vi "test TCX read (installed 71).vi"() -> ()   [LabVIEW 2011] (continued)
ackpoint><Time>2008-03-03T23:06:16Z</Time><Position><LatitudeDegrees>35.865661</LatitudeDegrees><LongitudeDegrees>-78.879918</LongitudeDegrees></Position><AltitudeMeters>73.678</AltitudeMeters><DistanceMeters>11620.606</DistanceMeters><Cadence>66</Cadence><Extensions><TPX xmlns=\"http://www.garmin.com/xmlschemas/ActivityExtension/v2\"><Watts>364</Watts></TPX></Extensions></Trackpoint><Trackpoint><Time>2008-03-03T23:06:17Z</Time><Position><LatitudeDegrees>35.865731</LatitudeDegrees><LongitudeDegrees>-78.879935</LongitudeDegrees></Position><AltitudeMeters>73.678</AltitudeMeters><DistanceMeters>11628.598</DistanceMeters><Cadence>65</Cadence><Extensions><TPX xmlns=\"http://www.garmin.com/xmlschemas/ActivityExtension/v2\"><Watts>362</Watts></TPX></Extensions></Trackpoint><Trackpoint><Time>2008-03-03T23:06:18Z</Time><Position><LatitudeDegrees>35.865801</LatitudeDegrees><LongitudeDegrees>-78.879955</LongitudeDegrees></Position><AltitudeMeters>73.678</AltitudeMeters><DistanceMeters>11636.497</DistanceMeters><Cadence>65</Cadence><Extensions><TPX xmlns=\"http://www.garmin.com/xmlschemas/ActivityExtension/v2\"><Watts>356</Watts></TPX></Extensions></Trackpoint><Trackpoint><Time>2008-03-03T23:06:19Z</Time><Position><LatitudeDegrees>35.865870</LatitudeDegrees><LongitudeDegrees>-78.879979</LongitudeDegrees></Position><AltitudeMeters>74.159</AltitudeMeters><DistanceMeters>11644.413</DistanceMeters><Cadence>65</Cadence><Extensions><TPX xmlns=\"http://www.garmin.com/xmlschemas/ActivityExtension/v2\"><Watts>355</Watts></TPX></Extensions></Trackpoint><Trackpoint><Time>2008-03-03T23:06:20Z</Time><Position><LatitudeDegrees>35.865936</LatitudeDegrees><LongitudeDegrees>-78.880009</LongitudeDegrees></Position><AltitudeMeters>74.640</AltitudeMeters><DistanceMeters>11652.265</DistanceMeters><Cadence>64</Cadence><Extensions><TPX xmlns=\"http://www.garmin.com/xmlschemas/ActivityExtension/v2\"><Watts>312</Watts></TPX></Extensions></Trackpoint><Trackpoint><Time>2008-03-03T23:06:21Z</Time><Position><LatitudeDegrees>35.866001</LatitudeDegrees><LongitudeDegrees>-78.880044</LongitudeDegrees></Position><AltitudeMeters>74.640</AltitudeMeters><DistanceMeters>11660.149</DistanceMeters><Cadence>64</Cadence><Extensions><TPX xmlns=\"http://www.garmin.com/xmlschemas/ActivityExtension/v2\"><Watts>275</Watts></TPX></Extensions></Trackpoint><Trackpoint><Time>2008-03-03T23:06:22Z</Time><Position><LatitudeDegrees>35.866066</LatitudeDegrees><LongitudeDegrees>-78.880082</LongitudeDegrees></Position><AltitudeMeters>74.640</AltitudeMeters><DistanceMeters>11668.127</DistanceMeters><Cadence>64</Cadence><Extensions><TPX xmlns=\"http://www.garmin.com/xmlschemas/ActivityExtension/v2\"><Watts>233</Watts></TPX></Extensions></Trackpoint><Trackpoint><Time>2008-03-03T23:06:23Z</Time><Position><LatitudeDegrees>35.866131</LatitudeDegrees><LongitudeDegrees>-78.880120</LongitudeDegrees></Position><AltitudeMeters>74.640</AltitudeMeters><DistanceMeters>11676.109</DistanceMeters><Cadence>65</Cadence><Extensions><TPX xmlns=\"http://www.garmin.com/xmlschemas/ActivityExtension/v2\"><Watts>109</Watts></TPX></Extensions></Trackpoint><Trackpoint><Time>2008-03-03T23:06:24Z</Time><Position><LatitudeDegrees>35.866196</LatitudeDegrees><LongitudeDegrees>-78.880160</LongitudeDegrees></Position><AltitudeMeters>74.640</AltitudeMeters><DistanceMeters>11684.144</DistanceMeters><Cadence>66</Cadence><Extensions><TPX xmlns=\"http://www.garmin.com/xmlschemas/ActivityExtension/v2\"><Watts>66</Watts></TPX></Extensions></Trackpoint><Trackpoint><Time>2008-03-03T23:06:25Z</Time><Position><LatitudeDegrees>35.866260</LatitudeDegrees><LongitudeDegrees>-78.880202</LongitudeDegrees></Position><AltitudeMeters>74.640</AltitudeMeters><DistanceMeters>11692.274</DistanceMeters><Cadence>66</Cadence><Extensions><TPX xmlns=\"http://www.garmin.com/xmlschemas/ActivityExtension/v2\"><Watts>59</Watts></TPX></Extensions></Trackpoint><Trackpoint><Time>2008-03-03T23:06:26Z</Time><Position><LatitudeDegrees>35.866323</LatitudeDegrees><LongitudeDegrees>-78.880250</LongitudeDegrees></Position><AltitudeMeters>74.640</AltitudeMeters><DistanceMeters>11700.427</DistanceMeters><Cadence>66</Cadence><Extensions><TPX xmlns=\"http://www.garmin.com/xmlschemas/ActivityExtension/v2\"><Watts>59</Watts></TPX></Extensions></Trackpoint><Trackpoint><Time>2008-03-03T23:06:27Z</Time><Position><LatitudeDegrees>35.866380</LatitudeDegrees><LongitudeDegrees>-78.880308</LongitudeDegrees></Position><AltitudeMeters>74.640</AltitudeMeters><DistanceMeters>11708.690</DistanceMeters><Cadence>68</Cadence><Extensions><TPX xmlns=\"http://www.garmin.com/xmlschemas/ActivityExtension/v2\"><Watts>59</Watts></TPX></Extensions></Trackpoint><Trackpoint><Time>2008-03-03T23:06:28Z</Time><Position><LatitudeDegrees>35.866422</LatitudeDegrees><LongitudeDegrees>-78.880383</LongitudeDegrees></Position><AltitudeMeters>74.640</AltitudeMeters><DistanceMeters>11716.855</DistanceMeters><Cadence>71</Cadence><Extensions><TPX xmlns=\"http://www.garmin.com/xmlschemas/ActivityExtension/v2\"><Watts>97</Watts></TPX></Extensions></Trackpoint><Trackpoint><Time>2008-03-03T23:06:29Z</Time><Position><LatitudeDegrees>35.866438</LatitudeDegrees><LongitudeDegrees>-78.880474</LongitudeDegrees></Position><AltitudeMeters>75.120</AltitudeMeters><DistanceMeters>11725.147</DistanceMeters><Cadence>71</Cadence><Extensions><TPX xmlns=\"http://www.garmin.com/xmlschemas/ActivityExtension/v2\"><Watts>97</Watts></TPX></Extensions></Trackpoint><Trackpoint><Time>2008-03-03T23:06:30Z</Time><Position><LatitudeDegrees>35.866425</LatitudeDegrees><LongitudeDegrees>-78.880568</LongitudeDegrees></Position><AltitudeMeters>74.640</AltitudeMeters><DistanceMeters>11733.718</DistanceMeters><Cadence>71</Cadence><Extensions><TPX xmlns=\"http://www.garmin.com/xmlschemas/ActivityExtension/v2\"><Watts>199</Watts></TPX></Extensions></Trackpoint><Trackpoint><Time>2008-03-03T23:06:31Z</Time><Position><LatitudeDegrees>35.866393</LatitudeDegrees><LongitudeDegrees>-78.880658</LongitudeDegrees></Position><AltitudeMeters>74.640</AltitudeMeters><DistanceMeters>11742.621</DistanceMeters><Cadence>71</Cadence><Extensions><TPX xmlns=\"http://www.garmin.com/xmlschemas/ActivityExtension/v2\"><Watts>199</Watts></TPX></Extensions></Trackpoint><Trackpoint><Time>2008-03-03T23:06:32Z</Time><Position><LatitudeDegrees>35.866355</LatitudeDegrees><LongitudeDegrees>-78.880747</LongitudeDegrees></Position><AltitudeMeters>75.120</AltitudeMeters><DistanceMeters>11751.724</DistanceMeters><Cadence>73</Cadence><Extensions><TPX xmlns=\"http://www.garmin.com/xmlschemas/ActivityExtension/v2\"><Watts>228</Watts></TPX></Extensions></Trackpoint><Trackpoint><Time>2008-03-03T23:06:33Z</Time><Position><LatitudeDegrees>35.866317</LatitudeDegrees><LongitudeDegrees>-78.880838</LongitudeDegrees></Position><AltitudeMeters>75.120</AltitudeMeters><DistanceMeters>11760.945</DistanceMeters><Cadence>75</Cadence><Extensions><TPX xmlns=\"http://www.garmin.com/xmlschemas/ActivityExtension/v2\"><Watts>280</Watts></TPX></Extensions></Trackpoint><Trackpoint><Time>2008-03-03T23:06:34Z</Time><Position><LatitudeDegrees>35.866279</LatitudeDegrees><LongitudeDegrees>-78.880931</LongitudeDegrees></Position><AltitudeMeters>75.120</AltitudeMeters><DistanceMeters>11770.377</DistanceMeters><Cadence>76</Cadence><Extensions><TPX xmlns=\"http://www.garmin.com/xmlschemas/ActivityExtension/v2\"><Watts>320</Watts></TPX></Extensions></Trackpoint><Trackpoint><Time>2008-03-03T23:06:35Z</Time><Position><LatitudeDegrees>35.866240</LatitudeDegrees><LongitudeDegrees>-78.881024</LongitudeDegrees></Position><AltitudeMeters>75.120</AltitudeMeters><DistanceMeters>11779.813</DistanceMeters><Cadence>76</Cadence><Extensions><TPX xmlns=\"http://www.garmin.com/xmlschemas/ActivityExtension/v2\"><Watts>272</Watts></TPX></Extensions></Trackpoint><Trackpoint><Time>2008-03-03T23:06:36Z</Time><Position><LatitudeDegrees>35.866200</LatitudeDegrees><LongitudeDegrees>-78.881116</LongitudeDegrees></Position><AltitudeMeters>75.120</AltitudeMeters><DistanceMeters>11789.220</DistanceMeters><Cadence>76</Cadence><Extensions><TPX xmlns=\"http://www.garmin.com/xmlschemas/ActivityExtension/v2\"><Watts>270</Watts></TPX></Extensions></Trackpoint><Trackpoint><Time>2008-03-03T23:06:37Z</Time><Position><LatitudeDegrees>35.866164</LatitudeDegrees><LongitudeDegrees>-78.881205</LongitudeDegrees></Position><AltitudeMeters>75.120</AltitudeMeters><DistanceMeters>11798.199</DistanceMeters><Cadence>75</Cadence><Extensions><TPX xmlns=\"http://www.garmin.com/xmlschemas/ActivityExtension/v2\"><Watts>204</Watts></TPX></Extensions></Trackpoint><Trackpoint><Time>2008-03-03T23:06:38Z</Time><Position><LatitudeDegrees>35.866129</LatitudeDegrees><LongitudeDegrees>-78.881295</LongitudeDegrees></Position><AltitudeMeters>75.601</AltitudeMeters><DistanceMeters>11807.172</DistanceMeters><Cadence>73</Cadence><Extensions><TPX xmlns=\"http://www.garmin.com/xmlschemas/ActivityExtension/v2\"><Watts>205</Watts></TPX></Extensions></Trackpoint><Trackpoint><Time>2008-03-03T23:06:39Z</Time><Position><LatitudeDegrees>35.866092</LatitudeDegrees><LongitudeDegrees>-78.881383</LongitudeDegrees></Position><AltitudeMeters>75.601</AltitudeMeters><DistanceMeters>11816.092</DistanceMeters><Cadence>71</Cadence><Extensions><TPX xmlns=\"http://www.garmin.com/xmlschemas/ActivityExtension/v2\"><Watts>231</Watts></TPX></Extensions></Trackpoint><Trackpoint><Time>2008-03-03T23:06:40Z</Time><Position><LatitudeDegrees>35.866055</LatitudeDegrees><LongitudeDegrees>-78.881469</LongitudeDegrees></Position><AltitudeMeters>75.120</AltitudeMeters><DistanceMeters>11824.877</DistanceMeters><Cadence>70</Cadence><Extensions><TPX xmlns=\"http://www.garmin.com/xmlschemas/ActivityExtension/v2\"><Watts>239</Watts></TPX></Extensions></Trackpoint><Trackpoint><Time>2008-03-03T23:06:41Z</Time><Position><LatitudeDegrees>35.866018</LatitudeDegrees><LongitudeDegrees>-78.881553</LongitudeDegrees></Position><AltitudeMeters>75.601</AltitudeMeters><DistanceMeters>11833.483</DistanceMeters><Cadence>70</Cadence><Extensions><TPX xmlns=\"http://www.garmin.com/xmlschemas/ActivityExtension/v2\"><Watts>241</Watts></TPX></Extensions></Trackpoint><Trackpoint><Time>2008-03-03T23:06:42Z</Time><Position><LatitudeDegrees>35.865982</LatitudeDegrees><LongitudeDegrees>-78.881636</LongitudeDegrees></Position><AltitudeMeters>75.601</AltitudeMeters><DistanceMeters>11842.034</DistanceMeters><Cadence>69</Cadence><Extensions><TPX xmlns=\"http://www.garmin.com/xmlschemas/ActivityExtension/v2\"><Watts>250</Watts></TPX></Extensions></Trackpoint><Trackpoint><Time>2008-03-03T23:06:43Z</Time><Position><LatitudeDegrees>35.865947</LatitudeDegrees><LongitudeDegrees>-78.881719</LongitudeDegrees></Position><AltitudeMeters>76.081</AltitudeMeters><DistanceMeters>11850.508</DistanceMeters><Cadence>68</Cadence><Extensions><TPX xmlns=\"http://www.garmin.com/xmlschemas/ActivityExtension/v2\"><Watts>251</Watts></TPX></Extensions></Trackpoint><Trackpoint><Time>2008-03-03T23:06:44Z</Time><Position><LatitudeDegrees>35.865912</LatitudeDegrees><LongitudeDegrees>-78.881803</LongitudeDegrees></Position><AltitudeMeters>76.081</AltitudeMeters><DistanceMeters>11858.958</DistanceMeters><Cadence>68</Cadence><Extensions><TPX xmlns=\"http://www.garmin.com/xmlschemas/ActivityExtension/v2\"><Watts>243</Watts></TPX></Extensions></Trackpoint><Trackpoint><Time>2008-03-03T23:06:45Z</Time><Position><LatitudeDegrees>35.865877</LatitudeDegrees><LongitudeDegrees>-78.881885</LongitudeDegrees></Position><AltitudeMeters>76.081</AltitudeMeters><DistanceMeters>11867.346</DistanceMeters><Cadence>68</Cadence><Extensions><TPX xmlns=\"http://www.garmin.com/xmlschemas/ActivityExtension/v2\"><Watts>240</Watts></TPX></Extensions></Trackpoint><Trackpoint><Time>2008-03-03T23:06:46Z</Time><Position><LatitudeDegrees>35.865843</LatitudeDegrees><LongitudeDegrees>-78.881968</LongitudeDegrees></Position><AltitudeMeters>76.562</AltitudeMeters><DistanceMeters>11875.714</DistanceMeters><Cadence>67</Cadence><Extensions><TPX xmlns=\"http://www.garmin.com/xmlschemas/ActivityExtension/v2\"><Watts>234</Watts></TPX></Extensions></Trackpoint><Trackpoint><Time>2008-03-03T23:06:47Z</Time><Position><LatitudeDegrees>35.865810</LatitudeDegrees><LongitudeDegrees>-78.882051</LongitudeDegrees></Position><AltitudeMeters>76.562</AltitudeMeters><DistanceMeters>11884.056</DistanceMeters><Cadence>68</Cadence><Extensions><TPX xmlns=\"http://www.garmin.com/xmlschemas/ActivityExtension/v2\"><Watts>202</Watts></TPX></Extensions></Trackpoint><Trackpoint><Time>2008-03-03T23:06:48Z</Time><Position><LatitudeDegrees>35.865777</LatitudeDegrees><LongitudeDegrees>-78.882134</LongitudeDegrees></Position><AltitudeMeters>76.562</AltitudeMeters><DistanceMeters>11892.388</DistanceMeters><Cadence>68</Cadence><Extensions><TPX xmlns=\"http://www.garmin.com/xmlschemas/ActivityExtension/v2\"><Watts>201</Watts></TPX></Extensions></Trackpoint><Trackpoint><Time>2008-03-03T23:06:49Z</Time><Position><LatitudeDegrees>35.865744</LatitudeDegrees><LongitudeDegrees>-78.882217</LongitudeDegrees></Position><AltitudeMeters>77.043</AltitudeMeters><DistanceMeters>11900.713</DistanceMeters><Cadence>67</Cadence><Extensions><TPX xmlns=\"http://www.garmin.com/xmlschemas/ActivityExtension/v2\"><Watts>182</Watts></TPX></Extensions></Trackpoint><Trackpoint><Time>2008-03-03T23:06:50Z</Time><Position><LatitudeDegrees>35.865711</LatitudeDegrees><LongitudeDegrees>-78.882300</LongitudeDegrees></Position><AltitudeMeters>76.081</AltitudeMeters><DistanceMeters>11909.103</DistanceMeters><Cadence>68</Cadence><Extensions><TPX xmlns=\"http://www.garmin.com/xmlschemas/ActivityExtension/v2\"><Watts>153</Watts></TPX></Extensions></Trackpoint><Trackpoint><Time>2008-03-03T23:06:51Z</Time><Position><LatitudeDegrees>35.865679</LatitudeDegrees><LongitudeDegrees>-78.882385</LongitudeDegrees></Position><AltitudeMeters>77.043</AltitudeMeters><DistanceMeters>11917.494</DistanceMeters><Cadence>68</Cadence><Extensions><TPX xmlns=\"http://www.garmin.com/xmlschemas/ActivityExtension/v2\"><Watts>134</Watts></TPX></Extensions></Trackpoint><Trackpoint><Time>2008-03-03T23:06:52Z</Time><Position><LatitudeDegrees>35.865650</LatitudeDegrees><LongitudeDegrees>-78.882471</LongitudeDegrees></Position><AltitudeMeters>77.043</AltitudeMeters><DistanceMeters>11925.970</DistanceMeters><Cadence>69</Cadence><Extensions><TPX xmlns=\"http://www.garmin.com/xmlschemas/ActivityExtension/v2\"><Watts>120</Watts></TPX></Extensions></Trackpoint><Trackpoint><Time>2008-03-03T23:06:53Z</Time><Position><LatitudeDegrees>35.865621</LatitudeDegrees><LongitudeDegrees>-78.882559</LongitudeDegrees></Position><AltitudeMeters>76.562</AltitudeMeters><DistanceMeters>11934.501</DistanceMeters><Cadence>70</Cadence><Extensions><TPX xmlns=\"http://www.garmin.com/xmlschemas/ActivityExtension/v2\"><Watts>109</Watts></TPX></Extensions></Trackpoint><Trackpoint><Time>2008-03-03T23:06:54Z</Time><Position><LatitudeDegrees>35.865594</LatitudeDegrees><LongitudeDegrees>-78.882648</LongitudeDegrees></Position><AltitudeMeters>76.081</AltitudeMeters><DistanceMeters>11943.104</DistanceMeters><Cadence>70</Cadence><Extensions><TPX xmlns=\"http://www.garmin.com/xmlschemas/ActivityExtension/v2\"><Watts>103</Watts></TPX></Extensions></Trackpoint><Trackpoint><Time>2008-03-03T23:06:55Z</Time><Position><LatitudeDegrees>35.865566</LatitudeDegrees><LongitudeDegrees>-78.882738</LongitudeDegrees></Position><AltitudeMeters>76.081</AltitudeMeters><DistanceMeters>11951.811</DistanceMeters><Cadence>71</Cadence><Extensions><TPX xmlns=\"http://www.garmin.com/xmlschemas/ActivityExtension/v2\"><Watts>105</Watts></TPX></Extensions></Trackpoint><Trackpoint><Time>2008-03-03T23:06:56Z</Time><Position><LatitudeDegrees>35.865540</LatitudeDegrees><LongitudeDegrees>-78.882830</LongitudeDegrees></Position><AltitudeMeters>76.562</AltitudeMeters><DistanceMeters>11960.656</DistanceMeters><Cadence>71</Cadence><Extensions><TPX xmlns=\"http://www.garmin.com/xmlschemas/ActivityExtension/v2\"><Watts>104</Watts></TPX></Extensions></Trackpoint><Trackpoint><Time>2008-03-03T23:06:57Z</Time><Position><LatitudeDegrees>35.865514</LatitudeDegrees><LongitudeDegrees>-78.882923</LongitudeDegrees></Position><AltitudeMeters>76.081</AltitudeMeters><DistanceMeters>11969.581</DistanceMeters><Cadence>72</Cadence><Extensions><TPX xmlns=\"http://www.garmin.com/xmlschemas/ActivityExtension/v2\"><Watts>93</Watts></TPX></Extensions></Trackpoint><Trackpoint><Time>2008-03-03T23:06:58Z</Time><Position><LatitudeDegrees>35.865489</LatitudeDegrees><LongitudeDegrees>-78.883018</LongitudeDegrees></Position><AltitudeMeters>76.081</AltitudeMeters><DistanceMeters>11978.509</DistanceMeters><Cadence>72</Cadence><Extensions><TPX xmlns=\"http://www.garmin.com/xmlschemas/ActivityExtension/v2\"><Watts>76</Watts></TPX></Extensions></Trackpoint><Trackpoint><Time>2008-03-03T23:06:59Z</Time><Position><LatitudeDegrees>35.865465</LatitudeDegrees><LongitudeDegrees>-78.883113</LongitudeDegrees></Position><AltitudeMeters>76.562</AltitudeMeters><DistanceMeters>11987.519</DistanceMeters><Cadence>73</Cadence><Extensions><TPX xmlns=\"http://www.garmin.com/xmlschemas/ActivityExtension/v2\"><Watts>63</Watts></TPX></Extensions></Trackpoint><Trackpoint><Time>2008-03-03T23:07:00Z</Time><Position><LatitudeDegrees>35.865444</LatitudeDegrees><LongitudeDegrees>-78.883210</LongitudeDegrees></Position><AltitudeMeters>76.562</AltitudeMeters><DistanceMeters>11996.611</DistanceMeters><Cadence>74</Cadence><Extensions><TPX xmlns=\"http://www.garmin.com/xmlschemas/ActivityExtension/v2\"><Watts>55</Watts></TPX></Extensions></Trackpoint><Trackpoint><Time>2008-03-03T23:07:01Z</Time><Position><LatitudeDegrees>35.865422</LatitudeDegrees><LongitudeDegrees>-78.883308</LongitudeDegrees></Position><AltitudeMeters>75.601</AltitudeMeters><DistanceMeters>12005.785</DistanceMeters><Cadence>74</Cadence><Extensions><TPX xmlns=\"http://www.garmin.com/xmlschemas/ActivityExtension/v2\"><Watts>55</Watts></TPX></Extensions></Trackpoint><Trackpoint><Time>2008-03-03T23:07:02Z</Time><Position><LatitudeDegrees>35.865399</LatitudeDegrees><LongitudeDegrees>-78.883406</LongitudeDegrees></Position><AltitudeMeters>75.601</AltitudeMeters><DistanceMeters>12015.007</DistanceMeters><Cadence>0</Cadence></Trackpoint><Trackpoint><Time>2008-03-03T23:07:03Z</Time><Position><LatitudeDegrees>35.865377</LatitudeDegrees><LongitudeDegrees>-78.883504</LongitudeDegrees></Position><AltitudeMeters>75.601</AltitudeMeters><DistanceMeters>12024.128</DistanceMeters><Cadence>0</Cadence></Trackpoint><Trackpoint><Time>2008-03-03T23:07:04Z</Time><Position><LatitudeDegrees>35.865358</LatitudeDegrees><LongitudeDegrees>-78.883594</LongitudeDegrees></Position><AltitudeMeters>76.562</AltitudeMeters><DistanceMeters>12032.522</DistanceMeters><Cadence>0</Cadence></Trackpoint><Trackpoint><Time>2008-03-03T23:07:05Z</Time><Position><LatitudeDegrees>35.865340</LatitudeDegrees><LongitudeDegrees>-78.883675</LongitudeDegrees></Position><AltitudeMeters>76.562</AltitudeMeters><DistanceMeters>12040.042</DistanceMeters><Cadence>13</Cadence></Trackpoint><Trackpoint><Time>2008-03-03T23:07:06Z</Time><Position><LatitudeDegrees>35.865316</LatitudeDegrees><LongitudeDegrees>-78.883750</LongitudeDegrees></Position><AltitudeMeters>76.081</AltitudeMeters><DistanceMeters>12047.338</DistanceMeters><Cadence>59</Cadence><Extensions><TPX xmlns=\"http://www.garmin.com/xmlschemas/ActivityExtension/v2\"><Watts>75</Watts></TPX></Extensions></Trackpoint><Trackpoint><Time>2008-03-03T23:07:07Z</Time><Position><LatitudeDegrees>35.865275</LatitudeDegrees><LongitudeDegrees>-78.883815</LongitudeDegrees></Position><AltitudeMeters>75.601</AltitudeMeters><DistanceMeters>12054.691</DistanceMeters><Cadence>62</Cadence><Extensions><TPX xmlns=\"http://www.garmin.com/xmlschemas/ActivityExtension/v2\"><Watts>115</Watts></TPX></Extensions></Trackpoint><Trackpoint><Time>2008-03-03T23:07:08Z</Time><Position><LatitudeDegrees>35.865217</LatitudeDegrees><LongitudeDegrees>-78.883861</LongitudeDegrees></Position><AltitudeMeters>75.120</AltitudeMeters><DistanceMeters>12062.268</DistanceMeters><Cadence>62</Cadence><Extensions><TPX xmlns=\"http://www.garmin.com/xmlschemas/ActivityExtension/v2\"><Watts>114</Watts></TPX></Extensions></Trackpoint><Trackpoint><Time>2008-03-03T23:07:09Z</Time><Position><LatitudeDegrees>35.865149</LatitudeDegrees><LongitudeDegrees>-78.883879</LongitudeDegrees></Position><AltitudeMeters>74.640</AltitudeMeters><DistanceMeters>12069.919</DistanceMeters><Cadence>66</Cadence><Extensions><TPX xmlns=\"http://www.garmin.com/xmlschemas/ActivityExtension/v2\"><Watts>154</Watts></TPX></Extensions></Trackpoint><Trackpoint><Time>2008-03-03T23:07:10Z</Time><Position><LatitudeDegrees>35.865079</LatitudeDegrees><LongitudeDegrees>-78.883877</LongitudeDegrees></Position><AltitudeMeters>75.120</AltitudeMeters><DistanceMeters>12077.684</DistanceMeters><Cadence>71</Cadence><Extensions><TPX xmlns=\"http://www.garmin.com/xmlschemas/ActivityExtension/v2\"><Watts>192</Watts></TPX></Extensions></Trackpoint><Trackpoint><Time>2008-03-03T23:07:11Z</Time><Position><LatitudeDegrees>35.865009</LatitudeDegrees><LongitudeDegrees>-78.883869</LongitudeDegrees></Position><AltitudeMeters>75.601</AltitudeMeters><DistanceMeters>12085.451</DistanceMeters><Cadence>70</Cadence><Extensions><TPX xmlns=\"http://www.garmin.com/xmlschemas/ActivityExtension/v2\"><Watts>195</Watts></TPX></Extensions></Trackpoint><Trackpoint><Time>2008-03-03T23:07:12Z</Time><Position><LatitudeDegrees>35.864940</LatitudeDegrees><LongitudeDegrees>-78.883859</LongitudeDegrees></Position><AltitudeMeters>75.120</AltitudeMeters><DistanceMeters>12093.237</DistanceMeters><Cadence>70</Cadence><Extensions><TPX xmlns=\"http://www.garmin.com/xmlschemas/ActivityExtension/v2\"><Watts>227</Watts></TPX></Extensions></Trackpoint><Trackpoint><Time>2008-03-03T23:07:13Z</Time><Position><LatitudeDegrees>35.864871</LatitudeDegrees><LongitudeDegrees>-78.883848</LongitudeDegrees></Position><AltitudeMeters>75.601</AltitudeMeters><DistanceMeters>12100.943</DistanceMeters><Cadence>70</Cadence><Extensions><TPX xmlns=\"http://www.garmin.com/xmlschemas/ActivityExtension/v2\"><Watts>228</Watts></TPX></Extensions></Trackpoint><Trackpoint><Time>2008-03-03T23:07:14Z</Time><Position><LatitudeDegrees>35.864803</LatitudeDegrees><LongitudeDegrees>-78.883834</LongitudeDegrees></Position><AltitudeMeters>75.601</AltitudeMeters><DistanceMeters>12108.532</DistanceMeters><Cadence>70</Cadence><Extensions><TPX xmlns=\"http://www.garmin.com/xmlschemas/ActivityExtension/v2\"><Watts>274</Watts></TPX></Extensions></Trackpoint><Trackpoint><Time>2008-03-03T23:07:15Z</Time><Position><LatitudeDegrees>35.864735</LatitudeDegrees><LongitudeDegrees>-78.883821</LongitudeDegrees></Position><AltitudeMeters>75.120</AltitudeMeters><DistanceMeters>12116.174</DistanceMeters><Cadence>69</Cadence><Extensions><TPX xmlns=\"http://www.garmin.com/xmlschemas/ActivityExtension/v2\"><Watts>282</Watts></TPX></Extensions></Trackpoint><Trackpoint><Time>2008-03-03T23:07:16Z</Time><Position><LatitudeDegrees>35.864667</LatitudeDegrees><LongitudeDegrees>-78.883810</LongitudeDegrees></Position><AltitudeMeters>75.601</AltitudeMeters><DistanceMeters>12123.817</DistanceMeters><Cadence>68</Cadence><Extensions><TPX xmlns=\"http://www.garmin.com/xmlschemas/ActivityExtension/v2\"><Watts>277</Watts></TPX></Extensions></Trackpoint><Trackpoint><Time>2008-03-03T23:07:17Z</Time><Position><LatitudeDegrees>35.864600</LatitudeDegrees><LongitudeDegrees>-78.883799</LongitudeDegrees></Position><AltitudeMeters>76.081</AltitudeMeters><DistanceMeters>12131.279</DistanceMeters><Cadence>68</Cadence><Extensions><TPX xmlns=\"http://www.garmin.com/xmlschemas/ActivityExtension/v2\"><Watts>275</Watts></TPX></Extensions></Trackpoint><Trackpoint><Time>2008-03-03T23:07:18Z</Time><Position><LatitudeDegrees>35.864534</LatitudeDegrees><LongitudeDegrees>-78.883792</LongitudeDegrees></Position><AltitudeMeters>76.081</AltitudeMeters><DistanceMeters>12138.690</DistanceMeters><Cadence>68</Cadence><Extensions><TPX xmlns=\"http://www.garmin.com/xmlschemas/ActivityExtension/v2\"><Watts>275</Watts></TPX></Extensions></Trackpoint><Trackpoint><Time>2008-03-03T23:07:19Z</Time><Position><LatitudeDegrees>35.864469</LatitudeDegrees><LongitudeDegrees>-78.883785</LongitudeDegrees></Position><AltitudeMeters>76.081</AltitudeMeters><DistanceMeters>12145.921</DistanceMeters><Cadence>65</Cadence><Extensions><TPX xmlns=\"http://www.garmin.com/xmlschemas/ActivityExtension/v2\"><Watts>276</Watts></TPX></Extensions></Trackpoint><Trackpoint><Time>2008-03-03T23:07:20Z</Time><Position><LatitudeDegrees>35.864405</LatitudeDegrees><LongitudeDegrees>-78.883780</LongitudeDegrees></Position><AltitudeMeters>76.081</AltitudeMeters><DistanceMeters>12153.025</DistanceMeters><Cadence>65</Cadence><Extensions><TPX xmlns=\"http://www.garmin.com/xmlschemas/ActivityExtension/v2\"><Watts>275</Watts></TPX></Extensions></Trackpoint><Trackpoint><Time>2008-03-03T23:07:21Z</Time><Position><LatitudeDegrees>35.864341</LatitudeDegrees><LongitudeDegrees>-78.883777</LongitudeDegrees></Position><AltitudeMeters>76.562</AltitudeMeters><DistanceMeters>12160.106</DistanceMeters><Cadence>64</Cadence><Extensions><TPX xmlns=\"http://www.garmin.com/xmlschemas/ActivityExtension/v2\"><Watts>267</Watts></TPX></Extensions></Trackpoint><Trackpoint><Time>2008-03-03T23:07:22Z</Time><Position><LatitudeDegrees>35.864278</LatitudeDegrees><LongitudeDegrees>-78.883776</LongitudeDegrees></Position><AltitudeMeters>76.562</AltitudeMeters><DistanceMeters>12167.061</DistanceMeters><Cadence>64</Cadence><Extensions><TPX xmlns=\"http://www.garmin.com/xmlschemas/ActivityExtension/v2\"><Watts>250</Watts></TPX></Extensions></Trackpoint><Trackpoint><Time>2008-03-03T23:07:23Z</Time><Position><LatitudeDegrees>35.864216</LatitudeDegrees><LongitudeDegrees>-78.883775</LongitudeDegrees></Position><AltitudeMeters>76.562</AltitudeMeters><DistanceMeters>12173.911</DistanceMeters><Cadence>64</Cadence><Extensions><TPX xmlns=\"http://www.garmin.com/xmlschemas/ActivityExtension/v2\"><Watts>269</Watts></TPX></Extensions></Trackpoint><Trackpoint><Time>2008-03-03T23:07:24Z</Time><Position><LatitudeDegrees>35.864155</LatitudeDegrees><LongitudeDegrees>-78.883774</LongitudeDegrees></Position><AltitudeMeters>77.523</AltitudeMeters><DistanceMeters>12180.674</DistanceMeters><Cadence>62</Cadence><Extensions><TPX xmlns=\"http://www.garmin.com/xmlschemas/ActivityExtension/v2\"><Watts>251</Watts></TPX></Extensions></Trackpoint><Trackpoint><Time>2008-03-03T23:07:25Z</Time><Position><LatitudeDegrees>35.864096</LatitudeDegrees><LongitudeDegrees>-78.883774</LongitudeDegrees></Position><AltitudeMeters>78.004</AltitudeMeters><DistanceMeters>12187.282</DistanceMeters><Cadence>60</Cadence><Extensions><TPX xmlns=\"http://www.garmin.com/xmlschemas/ActivityExtension/v2\"><Watts>251</Watts></TPX></Extensions></Trackpoint><Trackpoint><Time>2008-03-03T23:07:26Z</Time><Position><LatitudeDegrees>35.864037</LatitudeDegrees><LongitudeDegrees>-78.883774</LongitudeDegrees></Position><AltitudeMeters>77.523</AltitudeMeters><DistanceMeters>12193.755</DistanceMeters><Cadence>59</Cadence><Extensions><TPX xmlns=\"http://www.garmin.com/xmlschemas/ActivityExtension/v2\"><Watts>272</Watts></TPX></Extensions></Trackpoint><Trackpoint><Time>2008-03-03T23:07:27Z</Time><Position><LatitudeDegrees>35.863979</LatitudeDegrees><LongitudeDegrees>-78.883776</LongitudeDegrees></Position><AltitudeMeters>78.004</AltitudeMeters><DistanceMeters>12200.217</DistanceMeters><Cadence>59</Cadence><Extensions><TPX xmlns=\"http://www.garmin.com/xmlschemas/ActivityExtension/v2\"><Watts>291</Watts></TPX></Extensions></Trackpoint><Trackpoint><Time>2008-03-03T23:07:28Z</Time><Position><LatitudeDegrees>35.863921</LatitudeDegrees><LongitudeDegrees>-78.883778</LongitudeDegrees></Position><AltitudeMeters>78.004</AltitudeMeters><DistanceMeters>12206.744</DistanceMeters><Cadence>60</Cadence><Extensions><TPX xmlns=\"http://www.garmin.com/xmlschemas/ActivityExtension/v2\"><Watts>288</Watts></TPX></Extensions></Trackpoint><Trackpoint><Time>2008-03-03T23:07:29Z</Time><Position><LatitudeDegrees>35.863861</LatitudeDegrees><LongitudeDegrees>-78.883781</LongitudeDegrees></Position><AltitudeMeters>78.004</AltitudeMeters><DistanceMeters>12213.327</DistanceMeters><Cadence>60</Cadence><Extensions><TPX xmlns=\"http://www.garmin.com/xmlschemas/ActivityExtension/v2\"><Watts>291</Watts></TPX></Extensions></Trackpoint><Trackpoint><Time>2008-03-03T23:07:30Z</Time><Position><LatitudeDegrees>35.863802</LatitudeDegrees><LongitudeDegrees>-78.883785</LongitudeDegrees></Position><AltitudeMeters>78.004</AltitudeMeters><DistanceMeters>12219.902</DistanceMeters><Cadence>60</Cadence><Extensions><TPX xmlns=\"http://www.garmin.com/xmlschemas/ActivityExtension/v2\"><Watts>262</Watts></TPX></Extensions></Trackpoint><Trackpoint><Time>2008-03-03T23:07:31Z</Time><Position><LatitudeDegrees>35.863743</LatitudeDegrees><LongitudeDegrees>-78.883789</LongitudeDegrees></Position><AltitudeMeters>78.004</AltitudeMeters><DistanceMeters>12226.460</DistanceMeters><Cadence>60</Cadence><Extensions><TPX xmlns=\"http://www.garmin.com/xmlschemas/ActivityExtension/v2\"><Watts>234</Watts></TPX></Extensions></Trackpoint><Trackpoint><Time>2008-03-03T23:07:32Z</Time><Position><LatitudeDegrees>35.863684</LatitudeDegrees><LongitudeDegrees>-78.883794</LongitudeDegrees></Position><AltitudeMeters>78.485</AltitudeMeters><DistanceMeters>12233.067</DistanceMeters><Cadence>61</Cadence><Extensions><TPX xmlns=\"http://www.garmin.com/xmlschemas/ActivityExtension/v2\"><Watts>229</Watts></TPX></Extensions></Trackpoint><Trackpoint><Time>2008-03-03T23:07:33Z</Time><Position><LatitudeDegrees>35.863624</LatitudeDegrees><LongitudeDegrees>-78.883801</LongitudeDegrees></Position><AltitudeMeters>78.965</AltitudeMeters><DistanceMeters>12239.708</DistanceMeters><Cadence>61</Cadence><Extensions><TPX xmlns=\"http://www.garmin.com/xmlschemas/ActivityExtension/v2\"><Watts>228</Watts></TPX></Extensions></Trackpoint><Trackpoint><Time>2008-03-03T23:07:34Z</Time><Position><LatitudeDegrees>35.863565</LatitudeDegrees><LongitudeDegrees>-78.883809</LongitudeDegrees></Position><AltitudeMeters>78.965</AltitudeMeters><DistanceMeters>12246.327</DistanceMeters><Cadence>61</Cadence><Extensions><TPX xmlns=\"http://www.garmin.com/xmlschemas/ActivityExtension/v2\"><Watts>216</Watts></TPX></Extensions></Trackpoint><Trackpoint><Time>2008-03-03T23:07:35Z</Time><Position><LatitudeDegrees>35.863505</LatitudeDegrees><LongitudeDegrees>-78.883818</LongitudeDegrees></Position><AltitudeMeters>78.965</AltitudeMeters><DistanceMeters>12252.950</DistanceMeters><Cadence>61</Cadence><Extensions><TPX xmlns=\"http://www.garmin.com/xmlschemas/ActivityExtension/v2\"><Watts>208</Watts></TPX></Extensions></Trackpoint><Trackpoint><Time>2008-03-03T23:07:36Z</Time><Position><LatitudeDegrees>35.863446</LatitudeDegrees><LongitudeDegrees>-78.883827</LongitudeDegrees></Position><AltitudeMeters>78.485</AltitudeMeters><DistanceMeters>12259.565</DistanceMeters><Cadence>61</Cadence><Extensions><TPX xmlns=\"http://www.garmin.com/xmlschemas/ActivityExtension/v2\"><Watts>203</Watts></TPX></Extensions></Trackpoint><Trackpoint><Time>2008-03-03T23:07:37Z</Time><Position><LatitudeDegrees>35.863386</LatitudeDegrees><LongitudeDegrees>-78.883837</LongitudeDegrees></Position><AltitudeMeters>78.485</AltitudeMeters><DistanceMeters>12266.303</DistanceMeters><Cadence>62</Cadence><Extensions><TPX xmlns=\"http://www.garmin.com/xmlschemas/ActivityExtension/v2\"><Watts>197</Watts></TPX></Extensions></Trackpoint><Trackpoint><Time>2008-03-03T23:07:38Z</Time><Position><LatitudeDegrees>35.863326</LatitudeDegrees><LongitudeDegrees>-78.883848</LongitudeDegrees></Position><AltitudeMeters>78.485</AltitudeMeters><DistanceMeters>12273.065</DistanceMeters><Cadence>62</Cadence><Extensions><TPX xmlns=\"http://www.garmin.com/xmlschemas/ActivityExtension/v2\"><Watts>193</Watts></TPX></Extensions></Trackpoint><Trackpoint><Time>2008-03-03T23:07:39Z</Time><Position><LatitudeDegrees>35.863265</LatitudeDegrees><LongitudeDegrees>-78.883859</LongitudeDegrees></Position><AltitudeMeters>79.446</AltitudeMeters><DistanceMeters>12279.868</DistanceMeters><Cadence>63</Cadence><Extensions><TPX xmlns=\"http://www.garmin.com/xmlschemas/ActivityExtension/v2\"><Watts>184</Watts></TPX></Extensions></Trackpoint><Trackpoint><Time>2008-03-03T23:07:40Z</Time><Position><LatitudeDegrees>35.863205</LatitudeDegrees><LongitudeDegrees>-78.883872</LongitudeDegrees></Position><AltitudeMeters>79.446</AltitudeMeters><DistanceMeters>12286.604</DistanceMeters><Cadence>63</Cadence><Extensions><TPX xmlns=\"http://www.garmin.com/xmlschemas/ActivityExtension/v2\"><Watts>183</Watts></TPX></Extensions></Trackpoint><Trackpoint><Time>2008-03-03T23:07:41Z</Time><Position><LatitudeDegrees>35.863147</LatitudeDegrees><LongitudeDegrees>-78.883892</LongitudeDegrees></Position><AltitudeMeters>78.965</AltitudeMeters><DistanceMeters>12293.334</DistanceMeters><Cadence>62</Cadence><Extensions><TPX xmlns=\"http://www.garmin.com/xmlschemas/ActivityExtension/v2\"><Watts>162</Watts></TPX></Extensions></Trackpoint><Trackpoint><Time>2008-03-03T23:07:42Z</Time><Position><LatitudeDegrees>35.863088</LatitudeDegrees><LongitudeDegrees>-78.883914</LongitudeDegrees></Position><AltitudeMeters>78.965</AltitudeMeters><DistanceMeters>12300.178</DistanceMeters><Cadence>63</Cadence><Extensions><TPX xmlns=\"http://www.garmin.com/xmlschemas/ActivityExtension/v2\"><Watts>147</Watts></TPX></Extensions></Trackpoint><Trackpoint><Time>2008-03-03T23:07:43Z</Time><Position><LatitudeDegrees>35.863028</LatitudeDegrees><LongitudeDegrees>-78.883936</LongitudeDegrees></Position><AltitudeMeters>78.965</AltitudeMeters><DistanceMeters>12307.153</DistanceMeters><Cadence>64</Cadence><Extensions><TPX xmlns=\"http://www.garmin.com/xmlschemas/ActivityExtension/v2\"><Watts>144</Watts></TPX></Extensions></Trackpoint><Trackpoint><Time>2008-03-03T23:07:44Z</Time><Position><LatitudeDegrees>35.862967</LatitudeDegrees><LongitudeDegrees>-78.883957</LongitudeDegrees></Position><AltitudeMeters>78.965</AltitudeMeters><DistanceMeters>12314.179</DistanceMeters><Cadence>65</Cadence><Extensions><TPX xmlns=\"http://www.garmin.com/xmlschemas/ActivityExtension/v2\"><Watts>142</Watts></TPX></Extensions></Trackpoint><Trackpoint><Time>2008-03-03T23:07:45Z</Time><Position><LatitudeDegrees>35.862905</LatitudeDegrees><LongitudeDegrees>-78.883978</LongitudeDegrees></Position><AltitudeMeters>78.965</AltitudeMeters><DistanceMeters>12321.257</DistanceMeters><Cadence>65</Cadence><Extensions><TPX xmlns=\"http://www.garmin.com/xmlschemas/ActivityExtension/v2\"><Watts>143</Watts></TPX></Extensions></Trackpoint><Trackpoint><Time>2008-03-03T23:07:46Z</Time><Position><LatitudeDegrees>35.862844</LatitudeDegrees><LongitudeDegrees>-78.884001</LongitudeDegrees></Position><AltitudeMeters>78.485</AltitudeMeters><DistanceMeters>12328.459</DistanceMeters><Cadence>66</Cadence><Extensions><TPX xmlns=\"http://www.garmin.com/xmlschemas/ActivityExtension/v2\"><Watts>140</Watts></TPX></Extensions></Trackpoint><Trackpoint><Time>2008-03-03T23:07:47Z</Time><Position><LatitudeDegrees>35.862781</LatitudeDegrees><LongitudeDegrees>-78.884022</LongitudeDegrees></Position><AltitudeMeters>78.485</AltitudeMeters><DistanceMeters>12335.673</DistanceMeters><Cadence>67</Cadence><Extensions><TPX xmlns=\"http://www.garmin.com/xmlschemas/ActivityExtension/v2\"><Watts>134</Watts></TPX></Extensions></Trackpoint><Trackpoint><Time>2008-03-03T23:07:48Z</Time><Position><LatitudeDegrees>35.862717</LatitudeDegrees><LongitudeDegrees>-78.884044</LongitudeDegrees></Position><AltitudeMeters>78.485</AltitudeMeters><DistanceMeters>12343.056</DistanceMeters><Cadence>68</Cadence><Extensions><TPX xmlns=\"http://www.garmin.com/xmlschemas/ActivityExtension/v2\"><Watts>109</Watts></TPX></Extensions></Trackpoint><Trackpoint><Time>2008-03-03T23:07:49Z</Time><Position><LatitudeDegrees>35.862653</LatitudeDegrees><LongitudeDegrees>-78.884068</LongitudeDegrees></Position><AltitudeMeters>78.965</AltitudeMeters><DistanceMeters>12350.438</DistanceMeters><Cadence>69</Cadence><Extensions><TPX xmlns=\"http://www.garmin.com/xmlschemas/ActivityExtension/v2\"><Watts>89</Watts></TPX></Extensions></Trackpoint><Trackpoint><Time>2008-03-03T23:07:50Z</Time><Position><LatitudeDegrees>35.862589</LatitudeDegrees><LongitudeDegrees>-78.884096</LongitudeDegrees></Position><AltitudeMeters>78.485</AltitudeMeters><DistanceMeters>12357.969</DistanceMeters><Cadence>69</Cadence><Extensions><TPX xmlns=\"http://www.garmin.com/xmlschemas/ActivityExtension/v2\"><Watts>89</Watts></TPX></Extensions></Trackpoint><Trackpoint><Time>2008-03-03T23:07:51Z</Time><Position><LatitudeDegrees>35.862525</LatitudeDegrees><LongitudeDegrees>-78.884125</LongitudeDegrees></Position><AltitudeMeters>78.965</AltitudeMeters><DistanceMeters>12365.548</DistanceMeters><Cadence>70</Cadence><Extensions><TPX xmlns=\"http://www.garmin.com/xmlschemas/ActivityExtension/v2\"><Watts>97</Watts></TPX></Extensions></Trackpoint><Trackpoint><Time>2008-03-03T23:07:52Z</Time><Position><LatitudeDegrees>35.862461</LatitudeDegrees><LongitudeDegrees>-78.884158</LongitudeDegrees></Position><AltitudeMeters>78.485</AltitudeMeters><DistanceMeters>12373.249</DistanceMeters><Cadence>70</Cadence><Extensions><TPX xmlns=\"http://www.garmin.com/xmlschemas/ActivityExtension/v2\"><Watts>96</Watts></TPX></Extensions></Trackpoint><Trackpoint><Time>2008-03-03T23:07:53Z</Time><Position><LatitudeDegrees>35.862398</LatitudeDegrees><LongitudeDegrees>-78.884194</LongitudeDegrees></Position><AltitudeMeters>78.004</AltitudeMeters><DistanceMeters>12381.042</DistanceMeters><Cadence>71</Cadence><Extensions><TPX xmlns=\"http://www.garmin.com/xmlschemas/ActivityExtension/v2\"><Watts>103</Watts></TPX></Extensions></Trackpoint><Trackpoint><Time>2008-03-03T23:07:54Z</Time><Position><LatitudeDegrees>35.862335</LatitudeDegrees><LongitudeDegrees>-78.884234</LongitudeDegrees></Position><AltitudeMeters>78.485</AltitudeMeters><DistanceMeters>12388.862</DistanceMeters><Cadence>72</Cadence><Extensions><TPX xmlns=\"http://www.garmin.com/xmlschemas/ActivityExtension/v2\"><Watts>89</Watts></TPX></Extensions></Trackpoint><Trackpoint><Time>2008-03-03T23:07:55Z</Time><Position><LatitudeDegrees>35.862272</LatitudeDegrees><LongitudeDegrees>-78.884276</LongitudeDegrees></Position><AltitudeMeters>78.004</AltitudeMeters><DistanceMeters>12396.826</DistanceMeters><Cadence>72</Cadence><Extensions><TPX xmlns=\"http://www.garmin.com/xmlschemas/ActivityExtension/v2\"><Watts>89</Watts></TPX></Extensions></Trackpoint><Trackpoint><Time>2008-03-03T23:07:56Z</Time><Position><LatitudeDegrees>35.862210</LatitudeDegrees><LongitudeDegrees>-78.884323</LongitudeDegrees></Position><AltitudeMeters>78.004</AltitudeMeters><DistanceMeters>12404.891</DistanceMeters><Cadence>74</Cadence><Extensions><TPX xmlns=\"http://www.garmin.com/xmlschemas/ActivityExtension/v2\"><Watts>75</Watts></TPX></Extensions></Trackpoint><Trackpoint><Time>2008-03-03T23:07:57Z</Time><Position><LatitudeDegrees>35.862149</LatitudeDegrees><LongitudeDegrees>-78.884372</LongitudeDegrees></Position><AltitudeMeters>78.004</AltitudeMeters><DistanceMeters>12412.932</DistanceMeters><Cadence>74</Cadence><Extensions><TPX xmlns=\"http://www.garmin.com/xmlschemas/ActivityExtension/v2\"><Watts>75</Watts></TPX></Extensions></Trackpoint><Trackpoint><Time>2008-03-03T23:07:58Z</Time><Position><LatitudeDegrees>35.862090</LatitudeDegrees><LongitudeDegrees>-78.884423</LongitudeDegrees></Position><AltitudeMeters>78.485</AltitudeMeters><DistanceMeters>12420.925</DistanceMeters><Cadence>73</Cadence><Extensions><TPX xmlns=\"http://www.garmin.com/xmlschemas/ActivityExtension/v2\"><Watts>74</Watts></TPX></Extensions></Trackpoint><Trackpoint><Time>2008-03-03T23:07:59Z</Time><Position><LatitudeDegrees>35.862032</LatitudeDegrees><LongitudeDegrees>-78.884474</LongitudeDegrees></Position><AltitudeMeters>78.004</AltitudeMeters><DistanceMeters>12428.931</DistanceMeters><Cadence>73</Cadence><Extensions><TPX xmlns=\"http://www.garmin.com/xmlschemas/ActivityExte
